vi "Teleop.vi"(10 "Match Info":T1={"Autonomous Elapsed Seconds"=0.0, "TeleOp Elapsed Seconds"=0.0, "Disabled Elapsed Seconds"=0.0, "Visited Autonomous"=FALSE, "Visited TeleOp"=FALSE, "Visited Disabled"=FALSE, "Autonomous Settings"={"Autonomous Style"=enum."Independent", "VI Refnum"=refnum}}, 11 "Call Context":T2) -> ()   [LabVIEW 2012]
doc: "This VI is called for each TeleOp packet received from the DS where the robot is not disabled. It is often used to read from the joysticks and update I/O or to update setpoints for timed control loops. It should complete and return within 20 milliseconds or it may miss DS packets."
uses:
  <vilib>/Rock Robotics/WPI/DriverStation/WPI_DriverStationDerivedRobotMode.ctl
  <vilib>/Rock Robotics/WPI/DriverStation/WPI_DriverStationMatch Info.ctl
  <vilib>/Rock Robotics/WPI/Relay/WPI_RelayValue.ctl
  Robot Global Data.vi
  <vilib>/Rock Robotics/WPI/Joystick/WPI_JoystickGetSetRefNum.vi
panel:
  out "Numeric 1":dbl(slide) scale=0.0..100.0
  out "Boolean 2":bool
  out "Boolean 1":bool
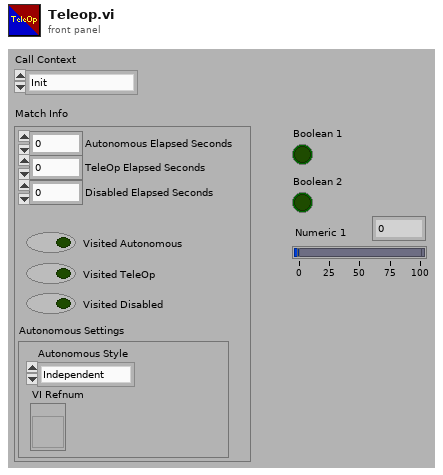
[diagram p1: front panel]
types:
  T1 = typedef "WPI_DriverStationMatch Info.ctl" = cluster{"Autonomous Elapsed Seconds":dbl, "TeleOp Elapsed Seconds":dbl, "Disabled Elapsed Seconds":dbl, "Visited Autonomous":bool, "Visited TeleOp":bool, "Visited Disabled":bool, "Autonomous Settings":cluster{"Autonomous Style":enum16{"Iterative", "Independent"}, "VI Refnum":refnum<vi>}}
  T2 = typedef "WPI_DriverStationDerivedRobotMode.ctl" = enum16{"Init", "Execute", "Stop"}
  T3 = typedef "WPI_RelayValue.ctl" = enum16{"Off", "On", "Forward", "Reverse"}
  T4 = typedef "WPI_RelayDevRef.ctl" = cluster{"DevStatus":errorcluster, "Relay Channel":T5, "Digital Module":T6, "Relay Direction":T7}
  T5 = typedef "FPGA_DIORelayChannel.ctl" = enum8{"Relay 1", "Relay 2", "Relay 3", "Relay 4", "Relay 5", "Relay 6", "Relay 7", "Relay 8", "Invalid"}
  T6 = typedef "FPGA_TypedefDigitalModule.ctl" = enum16{"Digital Module 1", "Digital Module 2"}
  T7 = typedef "WPI_RelayDirection.ctl" = enum16{"Both directions", "Forward only", "Reverse only"}
  T8 = typedef "WPI_JoystickDevRef.ctl" = cluster{"Device":T9}
  T9 = typedef "WPI_JoystickDeviceEnum.ctl" = enum16{"USB 1", "USB 2", "USB 3", "USB 4", "Kinect 1", "Kinect 2"}
  T10 = typedef "WPI_JoystickButtonState.ctl" = cluster{"Button 1":bool, "Button 2":bool, "Button 3":bool, "Button 4":bool, "Button 5":bool, "Button 6":bool, "Button 7":bool, "Button 8":bool, "Button 9":bool, "Button 10":bool, "Button 11":bool, "Button 12":bool}
  T11 = cluster{"axis 1 (x)":dbl, "axis 2 (y)":dbl, "axis 3 (throttle)":dbl, "axis 4":dbl, "axis 5":dbl, "axis 6":dbl}
  T12 = typedef "WPI_DigitalInputDevRef.ctl" = cluster{"DevStatus":errorcluster, "DIO Channel":T13, "Digital Module":T6}
  T13 = typedef "FPGA_DIOChannel.ctl" = enum8{"DIO 1", "DIO 2", "DIO 3", "DIO 4", "DIO 5", "DIO 6", "DIO 7", "DIO 8", "DIO 9", "DIO 10", "DIO 11", "DIO 12", "DIO 13", "DIO 14", "Invalid"}
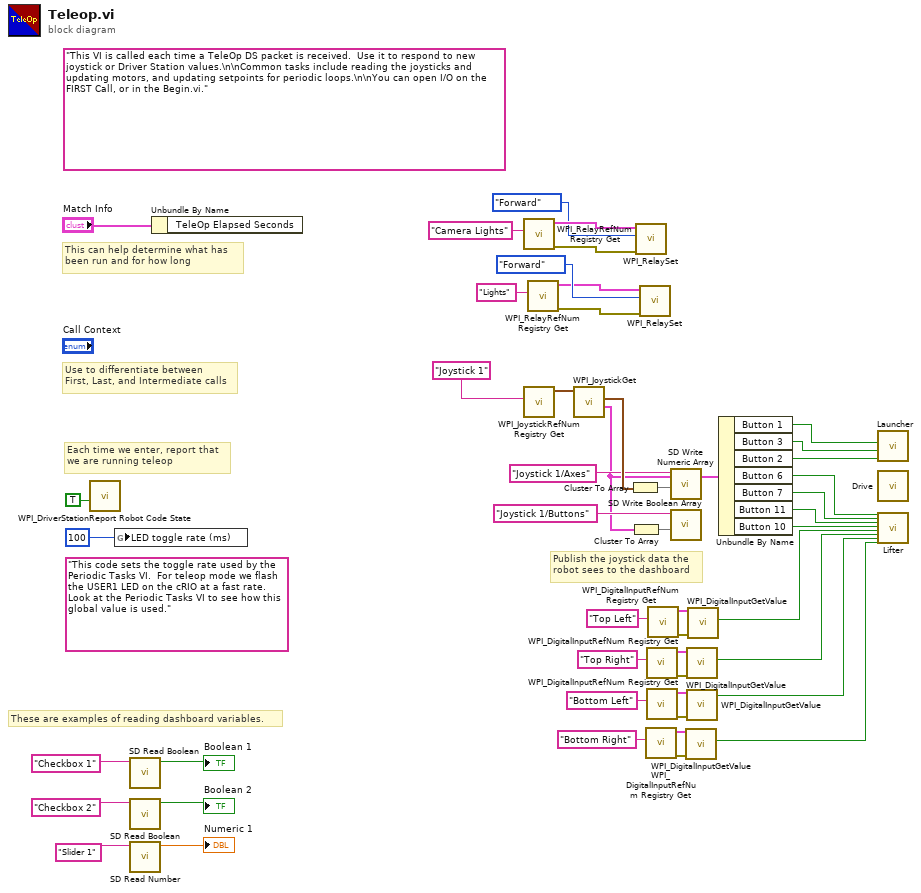
[diagram p0: block diagram]
diagram:
  (unwired) "This code sets the toggle rate used by the Periodic Tasks VI.  For teleop mode we flash the USER1 LED on the cRIO at a fast rate.  Look at the Periodic Tasks VI to see how this global value is used."
  (unwired) "This VI is called each time a TeleOp DS packet is received.  Use it to respond to new joystick or Driver Station values.\n\nCommon tasks include reading the joysticks and updating motors, and updating setpoints for periodic loops.\n\nYou can open I/O on the FIRST Call, or in the Begin.vi."
  # "Publish the joystick data the\nrobot sees to the dashboard"
  # "These are examples of reading dashboard variables."
  # "Each time we enter, report that\nwe are running teleop"
  # "Use to differentiate between\nFirst, Last, and Intermediate calls"
  # "This can help determine what has\nbeen run and for how long"
  n1 = call <vilib>:"WPI_DriverStationReport Robot Code State.vi"("TeleOp"=TRUE ("Autonomous")) -> ()  [unwired: 10 in, 1 out]
  n2 = global write "Robot Global Data.vi" "LED toggle rate (ms)"(u32 100 ("LED ms toggle rate")) -> ()
  n3 = call <vilib>:"SD Read Boolean.vi"("Name"="Checkbox 1" ("refnum name")) -> ("Boolean"=→"Boolean 1":bool)  [unwired: 8 in, 2 out]
  n4 = call <vilib>:"SD Read Boolean.vi"("Name"="Checkbox 2" ("refnum name")) -> ("Boolean"=→"Boolean 2":bool)  [unwired: 8 in, 2 out]
  n5 = call <vilib>:"SD Read Number.vi"("Name"="Slider 1" ("refnum name")) -> ("Numeric"=→"Numeric 1":dbl)  [unwired: 8 in, 2 out]
  n6 = Unbundle By Name("Match Info") -> ()  [unwired: 1 out]
  n7 = call <vilib>:"WPI_RelayRefNum Registry Get.vi"("refnum name"="Camera Lights") -> ("error out"=w31:errorcluster, "RelayDevRef"=w30:T4)  [unwired: 9 in]
  n8 = call <vilib>:"WPI_JoystickRefNum Registry Get.vi"("refnum name"="Joystick 1") -> ("JoystickDevRef"=w38:T8)  [unwired: 1 in, 9 out]
  n9 = call <vilib>:"WPI_RelayRefNum Registry Get.vi"("refnum name"="Lights") -> ("error out"=w1:errorcluster, "RelayDevRef"=w2:T4)  [unwired: 9 in]
  n10 = call <vilib>:"WPI_JoystickGet.vi"("JoystickDevRef"=w38) -> ("Buttons"=w32:T10, "Axes"=w36:T11)  [unwired: 1 in, 4 out]
  n11 = Cluster To Array(cluster=w36) -> (array=w34:dbl[])
  n12 = Cluster To Array(cluster=w32) -> (array=w37:bool[])
  n13 = call <vilib>:"WPI_RelaySet.vi"("error in (no error)"=w31, "RelayValue"=WPI_RelayValue."Forward", "RelayDevRef"=w30) -> ()  [unwired: 7 in, 2 out]
  n14 = call <vilib>:"WPI_RelaySet.vi"("error in (no error)"=w1, "RelayValue"=WPI_RelayValue."Forward", "RelayDevRef"=w2) -> ()  [unwired: 7 in, 2 out]
  n15 = call <vilib>:"WPI_DigitalInputRefNum Registry Get.vi"("refnum name"="Bottom Right") -> ("error out"=w10:errorcluster, "DigitalInputDevRef"=w9:T12)  [unwired: 9 in]
  n16 = call <vilib>:"WPI_DigitalInputRefNum Registry Get.vi"("refnum name"="Top Right") -> ("error out"=w14:errorcluster, "DigitalInputDevRef"=w13:T12)  [unwired: 9 in]
  n17 = call <vilib>:"WPI_DigitalInputRefNum Registry Get.vi"("refnum name"="Bottom Left") -> ("error out"=w12:errorcluster, "DigitalInputDevRef"=w11:T12)  [unwired: 9 in]
  n18 = call <vilib>:"WPI_DigitalInputRefNum Registry Get.vi"("refnum name"="Top Left") -> ("error out"=w16:errorcluster, "DigitalInputDevRef"=w15:T12)  [unwired: 9 in]
  n19 = call <vilib>:"SD Write Numeric Array.vi"("Numeric Array"=w34, "Name"="Joystick 1/Axes") -> ()  [unwired: 8 in, 2 out]
  n20 = call <vilib>:"SD Write Boolean Array.vi"("Boolean Array"=w37, "Name"="Joystick 1/Buttons") -> ()  [unwired: 8 in, 2 out]
  n21 = call <vilib>:"WPI_DigitalInputGetValue.vi"("error in (no error)"=w10, "DigitalInputDevRef"=w9) -> ("Value"=w5:bool)  [unwired: 7 in, 2 out]
  n22 = call <vilib>:"WPI_DigitalInputGetValue.vi"("error in (no error)"=w14, "DigitalInputDevRef"=w13) -> ("Value"=w7:bool)  [unwired: 7 in, 2 out]
  n23 = call <vilib>:"WPI_DigitalInputGetValue.vi"("error in (no error)"=w12, "DigitalInputDevRef"=w11) -> ("Value"=w6:bool)  [unwired: 7 in, 2 out]
  n24 = call <vilib>:"WPI_DigitalInputGetValue.vi"("error in (no error)"=w16, "DigitalInputDevRef"=w15) -> ("Value"=w8:bool)  [unwired: 7 in, 2 out]
  n25 = Unbundle By Name(w32) -> ("Button 1"=w21:bool, "Button 3"=w22:bool, "Button 2"=w23:bool, "Button 6"=w26:bool, "Button 7"=w27:bool, "Button 11"=w25:bool, "Button 10"=w24:bool)
  n26 = call "Launcher.vi"("Quicklaunch (2)"=w23, "Launch Button (3)"=w22, "Launch Motors On (1)"=w21) -> ()  [unwired: 9 in]
  n27 = call "Drive.vi"() -> ()  [unwired: 12 in]
  n28 = call "Lifter.vi"("Button 6 up"=w26, "Button 7 down"=w27, "Button 11 up"=w25, "Button 10 down"=w24, "top left"=w8, "top right"=w7, "bottom left"=w6, "bottom right"=w5) -> ()  [unwired: 20 in]
